vi "STICK_house_debugOnly.vi"() -> ()   [LabVIEW 2014]
panel:
  out "P2":T1
  in  "IDA 0 [V]":dbl
  out "P1":T2
  out "error out":errorcluster
  out "8 wire data":u8
  in  "VISA resource name":refnum<visa-resource-name>
  out "Device ID":string
  in  "Stop Button":bool
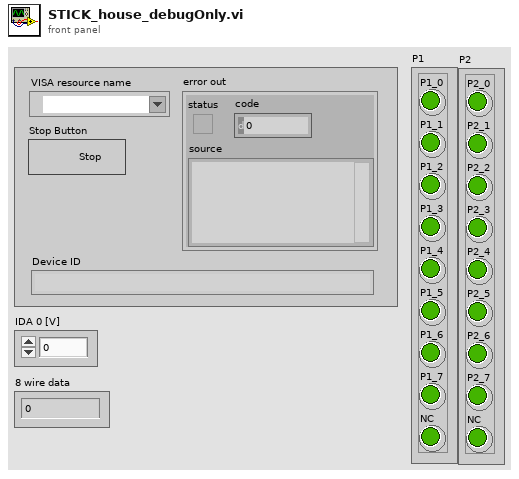
[diagram p1: front panel]
types:
  T1 = cluster{"P2_0":bool, "P2_1":bool, "P2_2":bool, "P2_3":bool, "P2_4":bool, "P2_5":bool, "P2_6":bool, "P2_7":bool, "NC":bool}
  T2 = cluster{"P1_0":bool, "P1_1":bool, "P1_2":bool, "P1_3":bool, "P1_4":bool, "P1_5":bool, "P1_6":bool, "P1_7":bool, "NC":bool}
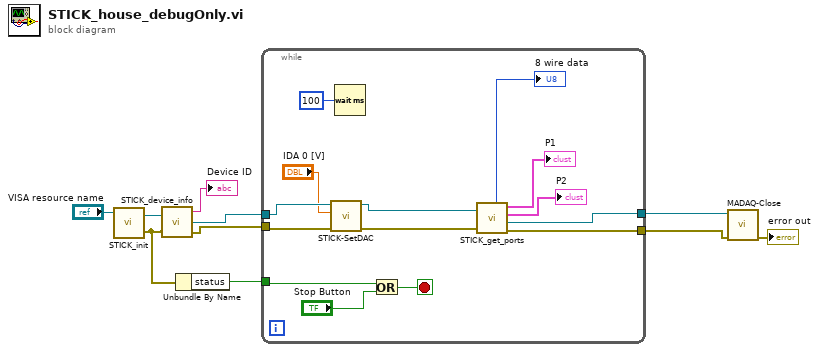
[diagram p0: block diagram]
diagram:
  n1 = call "STICK_init.vi"("VISA Refnum in"="VISA resource name") -> ("error out"=w4:errorcluster, "VISA Refnum out"=w5:refnum<visa-resource-name>)  [unwired: 1 in]
  n2 = call "STICK_device_info.vi"("VISA Refnum in"=w5, "error in (no error)"=w4) -> ("read buffer"=→"Device ID":string, "VISA Refnum out"=w2:refnum<visa-resource-name>, "error out"=w3:errorcluster)
  n3 = Unbundle By Name(w4) -> ("status"=w10:bool)
  n4 = while {
    tunnel: w10 -> [w17]
    tunnel: [w19] -> w7
    tunnel: [w18] -> w6
    tunnel: w3 -> [w15]
    tunnel: w2 -> [w16]
    stop <- w23 stop-if-true
    n5 = call "STICK-SetDAC.vi"("error in (no error)"=w15, "IDA 0 [V]"="IDA 0 [V]", "VISA resource name"=w16) -> ("error out"=w14:errorcluster, "VISA resource name out"=w13:refnum<visa-resource-name>)  [unwired: 3 in]
    n6 = Wait (ms)(milliseconds to wait=u32 100) -> ()  [unwired: 1 out]
    n7 = Or(x=w17, y="Stop Button") -> (x .or. y?=w23:bool)
    n8 = call "STICK_get_ports.vi"("error in (no error)"=w14, "VISA Refnum in"=w13) -> ("error out"=w18:errorcluster, "VISA Refnum out"=w19:refnum<visa-resource-name>, "P2"=→"P2":T1, "P1"=→"P1":T2, "data"=→"8 wire data":u8)
  }
  n9 = call "MADAQ-Close.vi"("error in (no error)"=w6, "VISA resource name"=w7) -> ("error out"=→"error out":errorcluster)  [unwired: 4 in, 1 out]
